vi "Read Data.vi"(5 "Address":T1 format="%02x", 6 "NoStop (F)":bool, 7 "I2C":refnum<class "I2C.lvclass">, 8 "error in (no error)":errorcluster, 9 "Len":u8, 11 "Session In":refnum<class "Session.lvclass">) -> (0 "error out":errorcluster, 1 "Data":string, 3 "Session Out":refnum<class "Session.lvclass">)   [LabVIEW 2024, in "CTI.lvlib" / "I2C.lvclass"]
uses:
  I2C.lvclass
  Session/Session.lvclass
  I2C Address.ctl
  I2C.lvclass/I2C.ctl
  CTI.lvlib
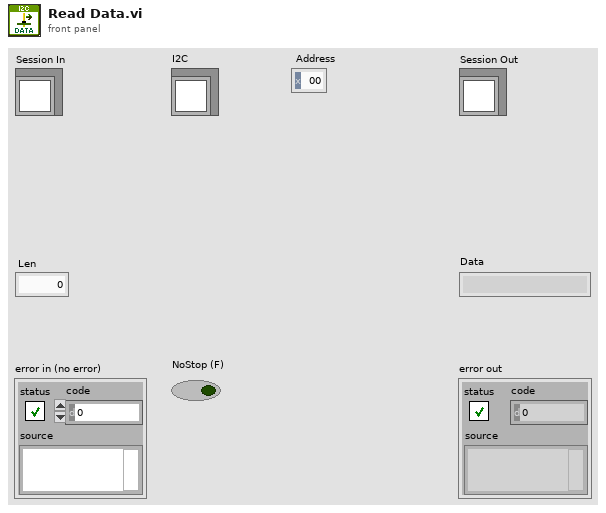
[diagram p1: front panel]
types:
  T1 = typedef "CTI.lvlib/I2C Address.ctl" = u8
  T2 = typedef "CTI.lvlib/I2C Number.ctl" = i8
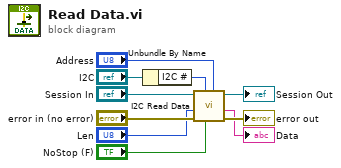
[diagram p0: block diagram]
diagram:
  n1 = Unbundle By Name("I2C") -> ("I2C #"=w2:T2)
  n2 = call "I2C Read Data.vi"("Address"="Address", "NoStop (F)"="NoStop (F)", "I2C #"=w2, "error in (no error)"="error in (no error)", "Len"="Len", "Session in"="Session In") -> ("error out"=→"error out":errorcluster, "Data"=→"Data":string, "Session out"=→"Session Out":refnum<class "Session.lvclass">)  [unwired: 3 in]
